vi "Read conn.vi"(8 "error in (no error)":errorcluster, 11 "instrXX in":refnum<class "instrXX.lvclass">) -> (0 "error out":errorcluster, 2 "conn":refnum<vi>, 3 "instrXX out":refnum<class "instrXX.lvclass">)   [LabVIEW 2017, in "instrXX.lvclass"]
uses:
  instrXX.lvclass
  instrXX.lvclass/instrXX.ctl
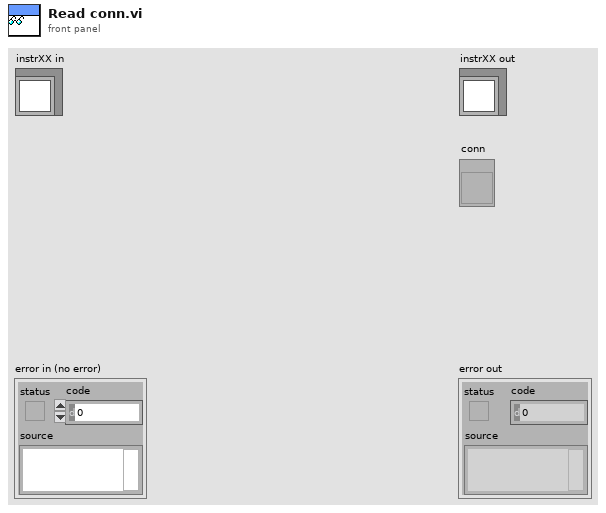
[diagram p1: front panel]
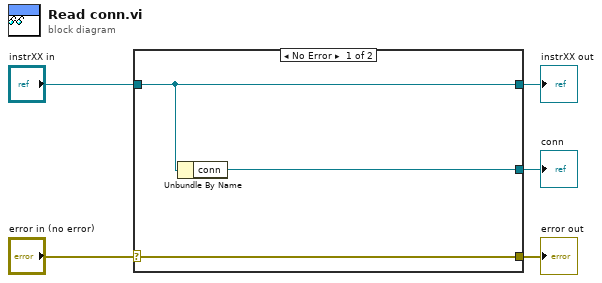
[diagram p0: block diagram]
diagram:
  n1 = case shown="No Error" "error in (no error)" {
    selector: "error in (no error)" -> [w8 w9]
    tunnel: [w8 w9] -> w4
    tunnel: [w7 w10] -> w2
    tunnel: "instrXX in" -> [w7 w10]
    tunnel: [w6 _] -> w1
    frame No Error {
      n2 = Unbundle By Name(w7) -> ("conn"=w6:refnum<vi>)
    }
    frame Error {
    }
  }
  "error out" <- w4
  "instrXX out" <- w2
  "conn" <- w1
